vi "read refnums.vi"(6 "call chain index (1)":i32=1, 7 "vi ref (caller)":refnum<vi>, 8 "error in (no error)":errorcluster, 11 "labels":string[](array[string])) -> (0 "error out":errorcluster, 3 "refnums":refnum<vi>[](array[refnum]))   [LabVIEW 2024, in "controls manager.lvlib"]
uses:
  controls manager.lvlib
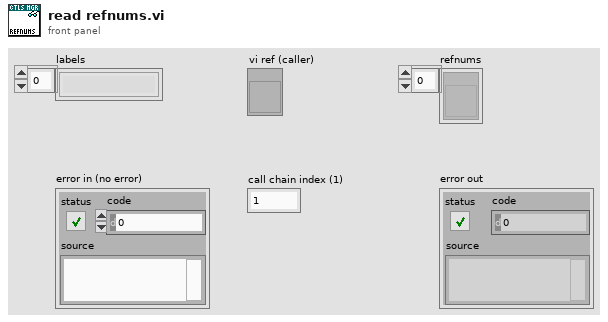
[diagram p1: front panel]
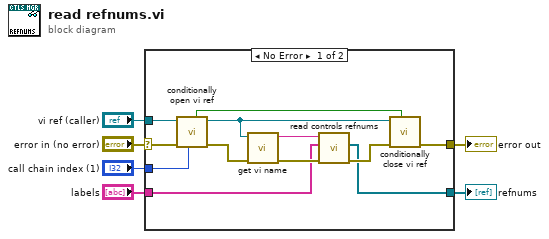
[diagram p0: block diagram]
diagram:
  n1 = case shown="No Error" "error in (no error)" {
    selector: "error in (no error)" -> [w17 w19]
    tunnel: [w14 w19] -> w6
    tunnel: "vi ref (caller)" -> [w11 _]
    tunnel: "call chain index (1)" -> [w10 _]
    tunnel: "labels" -> [w9 _]
    tunnel: [w8 _] -> w1
    frame No Error {
      n2 = call "conditionally open vi ref.vi"("call chain index (1)"=w10, "error in (no error)"=w17, "vi ref in"=w11) -> ("error out"=w16:errorcluster, "vi ref out"=w7:refnum<vi>, "new ref?"=w13:bool)  [unwired: 6 in]
      n3 = call "get vi name.vi"("error in (no error)"=w16, "vi ref"=w7) -> ("error out"=w18:errorcluster, "vi name"=w12:string)  [unwired: 8 in]
      n4 = call "read controls refnums.vi"("error in (no error)"=w18, "labels"=w9, "id"=w12) -> ("error out"=w15:errorcluster, "refnums"=w8:refnum<vi>[])  [unwired: 7 in]
      n5 = call "conditionally close vi ref.vi"("new ref?"=w13, "error in (no error)"=w15, "vi ref"=w7) -> ("error out"=w14:errorcluster)  [unwired: 8 in]
    }
    frame Error {
    }
  }
  "error out" <- w6
  "refnums" <- w1
